vi "Destroy User Event - Stop.vi"(8 "error in (no error)":errorcluster, 11 "user events in":T1) -> (0 "error out":errorcluster)   [LabVIEW 2019, in "User Events.lvlib"]
uses:
  User Events.lvlib
  emea-ni-adg-hla-lv/apps/generic/_typedefs/userEvents_type.ctl
  emea-ni-adg-hla-lv/apps/generic/_typedefs/app_data.ctl
  emea-ni-adg-hla-lv/src/helpers/Dictionaries/_typedefs/object_map_type.ctl
  emea-ni-adg-hla-lv/src/helpers/Dictionaries/_typedefs/object_type.ctl
  emea-ni-adg-hla-lv/src/helpers/Dictionaries/_typedefs/attribute_map_type.ctl
  emea-ni-adg-hla-lv/src/helpers/Dictionaries/_typedefs/attribute_type.ctl
  emea-ni-adg-hla-lv/src/helpers/Dictionaries/_typedefs/lv_dataType_type.ctl
  emea-ni-adg-hla-lv/src/helpers/Dictionaries/_typedefs/interaction_map_type.ctl
  emea-ni-adg-hla-lv/src/helpers/Dictionaries/_typedefs/interaction_type.ctl
  emea-ni-adg-hla-lv/src/helpers/Dictionaries/_typedefs/parameter_map_type.ctl
  emea-ni-adg-hla-lv/src/helpers/Dictionaries/_typedefs/parameter_type.ctl
  emea-ni-adg-hla-lv/src/helpers/Dictionaries/_typedefs/instanceHandle_map_type.ctl
  emea-ni-adg-hla-lv/src/helpers/ObjectManagement/ObjManager.lvlib
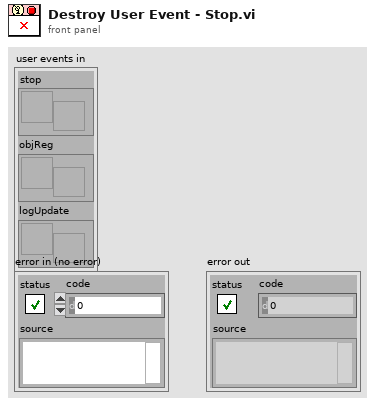
[diagram p1: front panel]
types:
  T1 = typedef "userEvents_type.ctl" = cluster{"stop":refnum<user-event>, "objReg":refnum<user-event>, "logUpdate":refnum<user-event>}
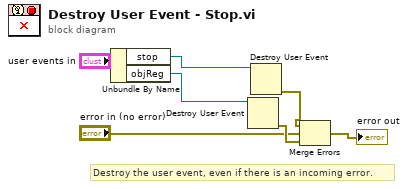
[diagram p0: block diagram]
diagram:
  # "Destroy the user event, even if there is an incoming error."
  n1 = Unbundle By Name("user events in") -> ("stop"=w2:refnum<user-event>, "objReg"=w1:refnum<user-event>)
  n2 = Destroy User Event(user event=w1) -> (error out=w7:errorcluster)  [unwired: 1 in]
  n3 = Destroy User Event(user event=w2) -> (error out=w4:errorcluster)  [unwired: 1 in]
  n4 = Merge Errors(w4, "error in (no error)", w7) -> (→"error out":errorcluster)
